vi "_Parse DBL Array Out Of Tolerance Result.vi"(8 "error in (no error)":errorcluster, 10 "Input String":string, 11 "VISA resource name":refnum<visa-resource-name>) -> (0 "error out":errorcluster, 1 "Results":dbl[](array[numeric]) format="%^.3e", 2 "Reliability":i32, 3 "VISA resource name out":refnum<visa-resource-name>, 5 "Out Of Tolerance":i32)   [LabVIEW 2015, in "Rohde&Schwarz CMP LR WPAN Measurement.lvlib"]
uses:
  <instrlib>/Rohde&Schwarz CMP LR WPAN Measurement/Rohde&Schwarz CMP LR WPAN Measurement.lvlib
  <instrlib>/Rohde&Schwarz CMP LR WPAN Measurement/Private/rsidr_core.llb/rsidr_core.lvlib
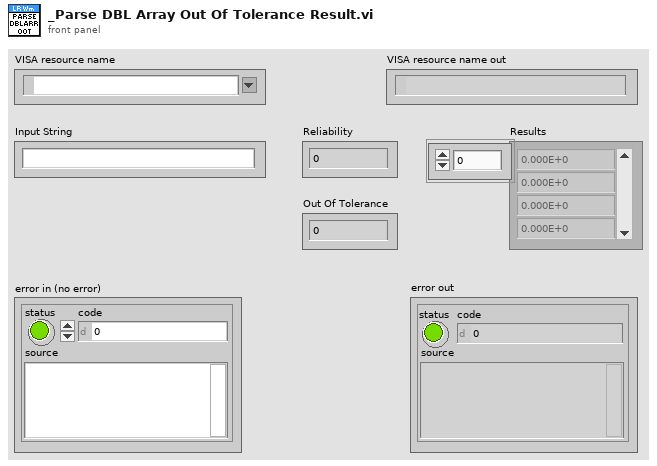
[diagram p1: front panel]
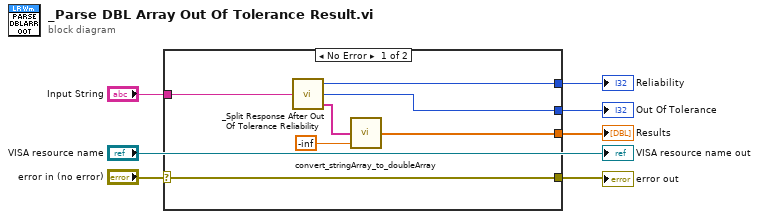
[diagram p0: block diagram]
diagram:
  n1 = case shown="No Error" "error in (no error)" {
    selector: "error in (no error)" -> [w9 w15]
    tunnel: [w12 _] -> w7
    tunnel: [w11 _] -> w6
    tunnel: [w10 _] -> w5
    tunnel: [w9 w15] -> w4
    tunnel: "Input String" -> [w8 _]
    frame No Error {
      n2 = call <instrlib>:"_Split Response After Out Of Tolerance Reliability.vi"("Input String"=w8) -> ("Reliability out"=w12:i32, "Out Of Tolerance"=w11:i32, "Response out"=w14:string[])
      n3 = call <instrlib>:"convert_stringArray_to_doubleArray.vi"("default (0)"=-inf ("Negative Infinity"), "string array in"=w14) -> ("double array out"=w10:dbl[])  [unwired: 3 in]
    }
    frame Error {
    }
  }
  "error out" <- w4
  "Reliability" <- w7
  "Results" <- w5
  "Out Of Tolerance" <- w6
  "VISA resource name out" <- "VISA resource name"
